vi "check_PVs_existed.vi"() -> ()   [LabVIEW 2013]
uses:
  <userlib>/caLab/Private/Get_PV-1D.vi
panel:
  out "Status":bool
  out "empty?":bool
  out "Numeric Control 2":i32
  out "1rst Value (string) 2":string[](array[string])
  out "Array 2":string[](array[string])
  out "Array":i32[](array[numeric])
  out "Numeric Control":i32
  out "sum":i16
  out "Error out":errorcluster
  out "size(s) 2":i32
  out "size(s)":i32
  out "1rst Value (string)":string[](array[string])
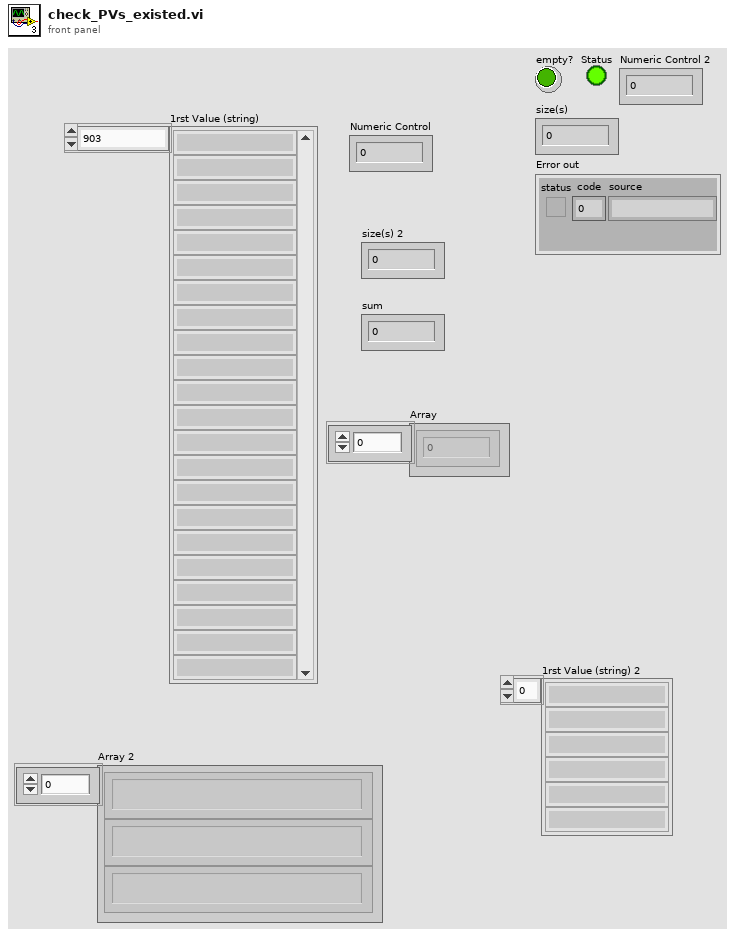
[diagram p1: front panel]
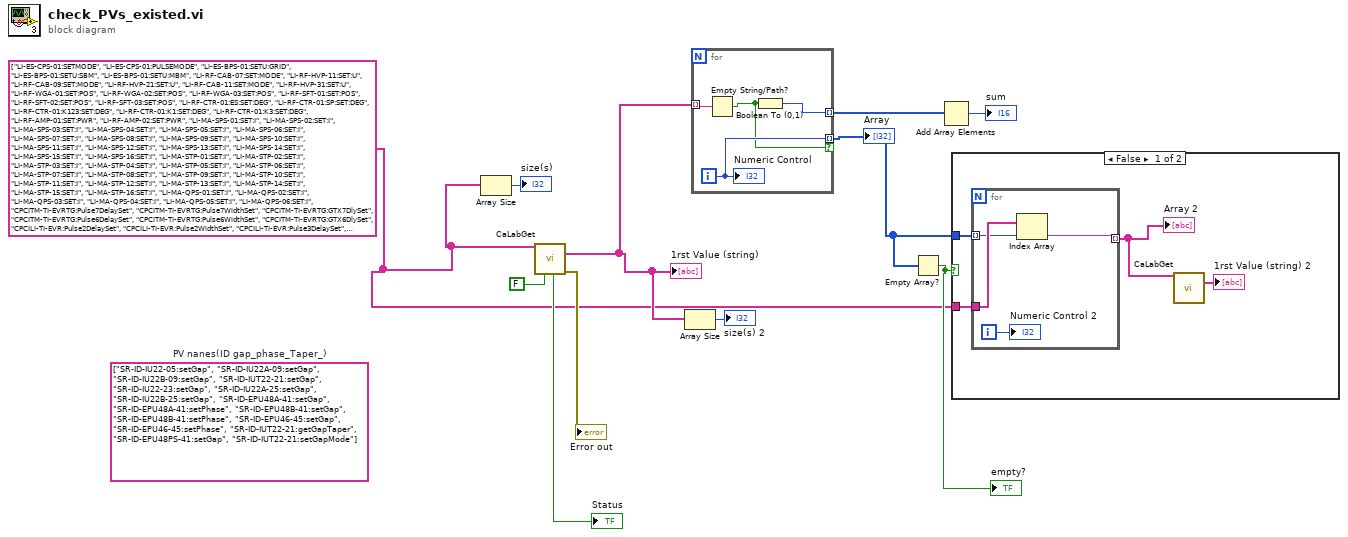
[diagram p0: block diagram]
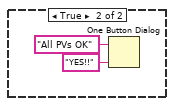
[diagram p2: hidden frame]
diagram:
  (unwired) string[] ["SR-ID-IU22-05:setGap", "SR-ID-IU22A-09:setGap", "SR-ID-IU22B-09:setGap", "SR-ID-IUT22-21:setGap", "SR-ID-IU22-23:setGap", "SR-ID-IU22A-25:setGap", "SR-ID-IU22B-25:setGap", "SR-ID-EPU48A-41:setGap", "SR-ID-EPU48A-41:setPhase", "SR-ID-EPU48B-41:setGap", "SR-ID-EPU48B-41:setPhase", "SR-ID-EPU46-45:setGap", "SR-ID-EPU46-45:setPhase", "SR-ID-IUT22-21:getGapTaper", "SR-ID-EPU48PS-41:setGap", "SR-ID-IUT22-21:setGapMode"]  # PV nanes(ID gap_phase_Taper_)
  w1 = string[] ["LI-ES-CPS-01:SETMODE", "LI-ES-CPS-01:PULSEMODE", "LI-ES-BPS-01:SETU:GRID", "LI-ES-BPS-01:SETU:SBM", "LI-ES-BPS-01:SETU:MBM", "LI-RF-CAB-07:SET:MODE", "LI-RF-HVP-11:SET:U", "LI-RF-CAB-09:SET:MODE", "LI-RF-HVP-21:SET:U", "LI-RF-CAB-11:SET:MODE", "LI-RF-HVP-31:SET:U", "LI-RF-WGA-01:SET:POS", "LI-RF-WGA-02:SET:POS", "LI-RF-WGA-03:SET:POS", "LI-RF-SFT-01:SET:POS", "LI-RF-SFT-02:SET:POS", "LI-RF-SFT-03:SET:POS", "LI-RF-CTR-01:ES:SET:DEG", "LI-RF-CTR-01:SP:SET:DEG", "LI-RF-CTR-01:K123:SET:DEG", "LI-RF-CTR-01:K1:SET:DEG", "LI-RF-CTR-01:K3:SET:DEG", "LI-RF-AMP-01:SET:PWR", "LI-RF-AMP-02:SET:PWR", "LI-MA-SPS-01:SET:I", "LI-MA-SPS-02:SET:I", "LI-MA-SPS-03:SET:I", "LI-MA-SPS-04:SET:I", "LI-MA-SPS-05:SET:I", "LI-MA-SPS-06:SET:I", "LI-MA-SPS-07:SET:I", "LI-MA-SPS-08:SET:I", "LI-MA-SPS-09:SET:I", "LI-MA-SPS-10:SET:I", "LI-MA-SPS-11:SET:I", "LI-MA-SPS-12:SET:I", "LI-MA-SPS-13:SET:I", "LI-MA-SPS-14:SET:I", "LI-MA-SPS-15:SET:I", "LI-MA-SPS-16:SET:I", "LI-MA-STP-01:SET:I", "LI-MA-STP-02:SET:I", "LI-MA-STP-03:SET:I", "LI-MA-STP-04:SET:I", "LI-MA-STP-05:SET:I", "LI-MA-STP-06:SET:I", "LI-MA-STP-07:SET:I", "LI-MA-STP-08:SET:I", "LI-MA-STP-09:SET:I", "LI-MA-STP-10:SET:I", "LI-MA-STP-11:SET:I", "LI-MA-STP-12:SET:I", "LI-MA-STP-13:SET:I", "LI-MA-STP-14:SET:I", "LI-MA-STP-15:SET:I", "LI-MA-STP-16:SET:I", "LI-MA-QPS-01:SET:I", "LI-MA-QPS-02:SET:I", "LI-MA-QPS-03:SET:I", "LI-MA-QPS-04:SET:I", "LI-MA-QPS-05:SET:I", "LI-MA-QPS-06:SET:I", "CPCITM-TI-EVRTG:Pulse7DelaySet", "CPCITM-TI-EVRTG:Pulse7WidthSet", "CPCITM-TI-EVRTG:GTX7DlySet", "CPCITM-TI-EVRTG:Pulse6DelaySet", "CPCITM-TI-EVRTG:Pulse6WidthSet", "CPCITM-TI-EVRTG:GTX6DlySet", "CPCILI-TI-EVR:Pulse2DelaySet", "CPCILI-TI-EVR:Pulse2WidthSet", "CPCILI-TI-EVR:Pulse3DelaySet", "CPCILI-TI-EVR:Pulse3WidthSet", "CPCILI-TI-EVR:Pulse4DelaySet", "CPCILI-TI-EVR:Pulse4WidthSet", "CPCILI-TI-EVR:Pulse5DelaySet", "CPCILI-TI-EVR:Pulse5WidthSet", "CPCILI-TI-EVR:Pulse6DelaySet", "CPCILI-TI-EVR:Pulse6WidthSet", "CPCILI-TI-EVR:Pulse7DelaySet", "CPCILI-TI-EVR:Pulse7WidthSet", "CPCILI-TI-EVR:Pulse8DelaySet", "CPCILI-TI-EVR:Pulse8WidthSet", "CPCILI-TI-EVR:Pulse9DelaySet", "CPCILI-TI-EVR:Pulse9WidthSet", "CPCITM-TI-EVRTG:GTX6DlySet", "CPCITM-TI-EVRTG:GTX7DlySet", "LTB-PS-HC-1:setI", "LTB-PS-HC-2:setI", "LTB-PS-HC-3:setI", "LTB-PS-HC-4:setI", "LTB-PS-HC-5:setI", "LTB-PS-VC-1:setI", "LTB-PS-VC-2:setI", "LTB-PS-VC-3:setI", "LTB-PS-VC-4:setI", "LTB-PS-VC-5:setI", "LTB-PS-VC-6:setI", "LTB-PS-VC-7:setI", "LTB-PS-Q1A:setI", "LTB-PS-Q1B:setI", "LTB-PS-Q1C:setI", "LTB-PS-Q2A:setI", "LTB-PS-Q2B:setI", "LTB-PS-Q2C:setI", "LTB-PS-Q3A:setI", "LTB-PS-Q3B:setI", "LTB-PS-Q4A:setI", "LTB-PS-Q4B:setI", "LTB-PS-QQ:setI", "LTB-PS-BEND-1:setI", "LTB-PS-VC-2a:setI", "LTB-PS-HC-3a:setI", "LTB-PS-HC-3b:setI", "LTB-PS-HC-4a:setI", "LTB-PS-HC-5a:setI", "LI-DI-SLIT-motor:axis2Position1", "LI-DI-SLIT-motor:axis1Position1", "BR-PS-HC-101:setI", "BR-PS-HC-102:setI", "BR-PS-HC-103:setI", "BR-PS-HC-104:setI", "BR-PS-HC-105:setI", "BR-PS-HC-106:setI", "BR-PS-HC-107:setI", "BR-PS-HC-108:setI", "BR-PS-HC-109:setI", "BR-PS-HC-110:setI", "BR-PS-HC-201:setI", "BR-PS-HC-202:setI", "BR-PS-HC-203:setI", "BR-PS-HC-204:setI", "BR-PS-HC-205:setI", "BR-PS-HC-206:setI", "BR-PS-HC-207:setI", "BR-PS-HC-208:setI", "BR-PS-HC-209:setI", "BR-PS-HC-210:setI", "BR-PS-HC-301:setI", "BR-PS-HC-302:setI", "BR-PS-HC-303:setI", "BR-PS-HC-304:setI", "BR-PS-HC-305:setI", "BR-PS-HC-306:setI", "BR-PS-HC-307:setI", "BR-PS-HC-308:setI", "BR-PS-HC-309:setI", "BR-PS-HC-310:setI", "BR-PS-HC-401:setI", "BR-PS-HC-402:setI", "BR-PS-HC-403:setI", "BR-PS-HC-404:setI", "BR-PS-HC-405:setI", "BR-PS-HC-406:setI", "BR-PS-HC-407:setI", "BR-PS-HC-408:setI", "BR-PS-HC-409:setI", "BR-PS-HC-410:setI", "BR-PS-HC-501:setI", "BR-PS-HC-502:setI", "BR-PS-HC-503:setI", "BR-PS-HC-504:setI", "BR-PS-HC-505:setI", "BR-PS-HC-506:setI", "BR-PS-HC-507:setI", "BR-PS-HC-508:setI", "BR-PS-HC-509:setI", "BR-PS-HC-510:setI", "BR-PS-HC-601:setI", "BR-PS-HC-602:setI", "BR-PS-HC-603:setI", "BR-PS-HC-603a:setI", "BR-PS-HC-604:setI", "BR-PS-HC-605:setI", "BR-PS-HC-606:setI", "BR-PS-HC-606a:setI", "BR-PS-HC-607:setI", "BR-PS-HC-608:setI", "BR-PS-HC-609:setI", "BR-PS-HC-610:setI", "BR-PS-VC-101:setI", "BR-PS-VC-102:setI", "BR-PS-VC-103:setI", "BR-PS-VC-104:setI", "BR-PS-VC-105:setI", "BR-PS-VC-106:setI", "BR-PS-VC-201:setI", "BR-PS-VC-202:setI", "BR-PS-VC-203:setI", "BR-PS-VC-204:setI", "BR-PS-VC-205:setI", "BR-PS-VC-206:setI", "BR-PS-VC-301:setI", "BR-PS-VC-302:setI", "BR-PS-VC-303:setI", "BR-PS-VC-304:setI", "BR-PS-VC-305:setI", "BR-PS-VC-306:setI", "BR-PS-VC-401:setI", "BR-PS-VC-402:setI", "BR-PS-VC-403:setI", "BR-PS-VC-404:setI", "BR-PS-VC-405:setI", "BR-PS-VC-406:setI", "BR-PS-VC-501:setI", "BR-PS-VC-502:setI", "BR-PS-VC-503:setI", "BR-PS-VC-504:setI", "BR-PS-VC-505:setI", "BR-PS-VC-506:setI", "BR-PS-VC-601:setI", "BR-PS-VC-602:setI", "BR-PS-VC-602a:setI", "BR-PS-VC-603:setI", "BR-PS-VC-604:setI", "BR-PS-VC-604a:setI", "BR-PS-VC-605:setI", "BR-PS-VC-606:setI", "BR-PS-VC-100a:setI", "BR-PS-SD:setI", "BR-PS-SF:setI", "cpsc_027:AO:SLOW_SET:CH:1", "cpsc_037:AO:SLOW_SET:CH:3", "BR-RF-LLRF:setStationPhase", "TI-INJ-PROC:setTinj", "BR-PS-INJ-SE:setHV", "CPCIPM-TI-EVR:Pulse1DelaySet", "BR-PS-INJ-KI:setHV", "CPCIPM-TI-EVR:Pulse2DelaySet", "BR-PS-QF:setWfDC", "BR-PS-QM:setWfDC", "BR-PS-Q1:setWfDC", "BR-PS-Q2:setWfDC", "BR-PS-BEND:setWfDC", "BTS-PS-HC-1:setI", "BTS-PS-HC-2:setI", "BTS-PS-HC-3:setI", "BTS-PS-HC-4:setI", "BTS-PS-HC-5:setI", "BTS-PS-VC-2:setI", "BTS-PS-VC-3:setI", "BTS-PS-VC-4:setI", "BTS-PS-VC-5:setI", "BTS-PS-VC-6:setI", "BTS-PS-Q1A:setI", "BTS-PS-Q1B:setI", "BTS-PS-Q1C:setI", "BTS-PS-Q2A:setI", "BTS-PS-Q2B:setI", "BTS-PS-Q2C:setI", "BTS-PS-Q3A:setI", "BTS-PS-BEND-1:setI", "BTS-PS-BEND-2:setI", "BR-PS-EXT-K1:setHV", "BR-PS-EXT-K2:setHV", "SR-PS-INJ-SE1:setHV", "SR-PS-INJ-SE2:setHV", "SR-PS-INJ-K1:setHV", "SR-PS-INJ-K2:setHV", "SR-PS-INJ-K3:setHV", "SR-PS-INJ-K4:setHV", "CPCIPM-TI-EVR:Pulse4DelaySet", "CPCIPM-TI-EVR:Pulse5DelaySet", "CPCIPM-TI-EVR:Pulse3DelaySet", "CPCIPM-TI-EVR:Pulse6DelaySet", "CPCIPM-TI-EVR:Pulse7DelaySet", "T560:setADelay", "T560:setBDelay", "T560:setCDelay", "T560:setDDelay", "CPCIPM-TI-EVR:Pulse4DelaySet", "CPCIPM-TI-EVR:Pulse5DelaySet", "BR-PS-EXT-SE1:setHV", "BR-PS-EXT-SE2:setHV", "CPCIPM-TI-EVR:Pulse3DelaySet", "CPCIPM-TI-EVR:Pulse11DelaySet", "SR-PS-BEND:setI", "SR-PS-HC-011:setI", "SR-PS-HC-012:setI", "SR-PS-HC-013:setI", "SR-PS-HC-014:setI", "SR-PS-HC-015:setI", "SR-PS-HC-016:setI", "SR-PS-HC-017:setI", "SR-PS-HC-021:setI", "SR-PS-HC-022:setI", "SR-PS-HC-023:setI", "SR-PS-HC-024:setI", "SR-PS-HC-025:setI", "SR-PS-HC-026:setI", "SR-PS-HC-027:setI", "SR-PS-HC-031:setI", "SR-PS-HC-032:setI", "SR-PS-HC-033:setI", "SR-PS-HC-034:setI", "SR-PS-HC-035:setI", "SR-PS-HC-036:setI", "SR-PS-HC-037:setI", "SR-PS-HC-041:setI", "SR-PS-HC-042:setI", "SR-PS-HC-043:setI", "SR-PS-HC-044:setI", "SR-PS-HC-045:setI", "SR-PS-HC-046:setI", "SR-PS-HC-047:setI", "SR-PS-HC-051:setI", "SR-PS-HC-052:setI", "SR-PS-HC-053:setI", "SR-PS-HC-054:setI", "SR-PS-HC-055:setI", "SR-PS-HC-056:setI", "SR-PS-HC-057:setI", "SR-PS-HC-061:setI", "SR-PS-HC-062:setI", "SR-PS-HC-063:setI", "SR-PS-HC-064:setI", "SR-PS-HC-065:setI", "SR-PS-HC-066:setI", "SR-PS-HC-067:setI", "SR-PS-HC-071:setI", "SR-PS-HC-072:setI", "SR-PS-HC-073:setI", "SR-PS-HC-074:setI", "SR-PS-HC-075:setI", "SR-PS-HC-076:setI", "SR-PS-HC-077:setI", "SR-PS-HC-081:setI", "SR-PS-HC-082:setI", "SR-PS-HC-083:setI", "SR-PS-HC-084:setI", "SR-PS-HC-085:setI", "SR-PS-HC-086:setI", "SR-PS-HC-087:setI", "SR-PS-HC-091:setI", "SR-PS-HC-092:setI", "SR-PS-HC-093:setI", "SR-PS-HC-094:setI", "SR-PS-HC-095:setI", "SR-PS-HC-096:setI", "SR-PS-HC-097:setI", "SR-PS-HC-101:setI", "SR-PS-HC-102:setI", "SR-PS-HC-103:setI", "SR-PS-HC-104:setI", "SR-PS-HC-105:setI", "SR-PS-HC-106:setI", "SR-PS-HC-107:setI", "SR-PS-HC-111:setI", "SR-PS-HC-112:setI", "SR-PS-HC-113:setI", "SR-PS-HC-114:setI", "SR-PS-HC-115:setI", "SR-PS-HC-116:setI", "SR-PS-HC-117:setI", "SR-PS-HC-121:setI", "SR-PS-HC-122:setI", "SR-PS-HC-123:setI", "SR-PS-HC-124:setI", "SR-PS-HC-125:setI", "SR-PS-HC-126:setI", "SR-PS-HC-127:setI", "SR-PS-HC-131:setI", "SR-PS-HC-132:setI", "SR-PS-HC-133:setI", "SR-PS-HC-134:setI", "SR-PS-HC-135:setI", "SR-PS-HC-136:setI", "SR-PS-HC-137:setI", "SR-PS-HC-141:setI", "SR-PS-HC-142:setI", "SR-PS-HC-143:setI", "SR-PS-HC-144:setI", "SR-PS-HC-145:setI", "SR-PS-HC-146:setI", "SR-PS-HC-147:setI", "SR-PS-HC-151:setI", "SR-PS-HC-152:setI", "SR-PS-HC-153:setI", "SR-PS-HC-154:setI", "SR-PS-HC-155:setI", "SR-PS-HC-156:setI", "SR-PS-HC-157:setI", "SR-PS-HC-161:setI", "SR-PS-HC-162:setI", "SR-PS-HC-163:setI", "SR-PS-HC-164:setI", "SR-PS-HC-165:setI", "SR-PS-HC-166:setI", "SR-PS-HC-167:setI", "SR-PS-HC-171:setI", "SR-PS-HC-172:setI", "SR-PS-HC-173:setI", "SR-PS-HC-174:setI", "SR-PS-HC-175:setI", "SR-PS-HC-176:setI", "SR-PS-HC-177:setI", "SR-PS-HC-181:setI", "SR-PS-HC-182:setI", "SR-PS-HC-183:setI", "SR-PS-HC-184:setI", "SR-PS-HC-185:setI", "SR-PS-HC-186:setI", "SR-PS-HC-187:setI", "SR-PS-HC-191:setI", "SR-PS-HC-192:setI", "SR-PS-HC-193:setI", "SR-PS-HC-194:setI", "SR-PS-HC-195:setI", "SR-PS-HC-196:setI", "SR-PS-HC-197:setI", "SR-PS-HC-201:setI", "SR-PS-HC-202:setI", "SR-PS-HC-203:setI", "SR-PS-HC-204:setI", "SR-PS-HC-205:setI", "SR-PS-HC-206:setI", "SR-PS-HC-207:setI", "SR-PS-HC-211:setI", "SR-PS-HC-212:setI", "SR-PS-HC-213:setI", "SR-PS-HC-214:setI", "SR-PS-HC-215:setI", "SR-PS-HC-216:setI", "SR-PS-HC-217:setI", "SR-PS-HC-221:setI", "SR-PS-HC-222:setI", "SR-PS-HC-223:setI", "SR-PS-HC-224:setI", "SR-PS-HC-225:setI", "SR-PS-HC-226:setI", "SR-PS-HC-227:setI", "SR-PS-HC-231:setI", "SR-PS-HC-232:setI", "SR-PS-HC-233:setI", "SR-PS-HC-234:setI", "SR-PS-HC-235:setI", "SR-PS-HC-236:setI", "SR-PS-HC-237:setI", "SR-PS-HC-241:setI", "SR-PS-HC-242:setI", "SR-PS-HC-243:setI", "SR-PS-HC-244:setI", "SR-PS-HC-245:setI", "SR-PS-HC-246:setI", "SR-PS-HC-247:setI", "SR-PS-VC-011:setI", "SR-PS-VC-012:setI", "SR-PS-VC-013:setI", "SR-PS-VC-014:setI", "SR-PS-VC-015:setI", "SR-PS-VC-016:setI", "SR-PS-VC-017:setI", "SR-PS-VC-021:setI", "SR-PS-VC-022:setI", "SR-PS-VC-023:setI", "SR-PS-VC-024:setI", "SR-PS-VC-025:setI", "SR-PS-VC-026:setI", "SR-PS-VC-027:setI", "SR-PS-VC-031:setI", "SR-PS-VC-032:setI", "SR-PS-VC-033:setI", "SR-PS-VC-034:setI", "SR-PS-VC-035:setI", "SR-PS-VC-036:setI", "SR-PS-VC-037:setI", "SR-PS-VC-041:setI", "SR-PS-VC-042:setI", "SR-PS-VC-043:setI", "SR-PS-VC-044:setI", "SR-PS-VC-045:setI", "SR-PS-VC-046:setI", "SR-PS-VC-047:setI", "SR-PS-VC-051:setI", "SR-PS-VC-052:setI", "SR-PS-VC-053:setI", "SR-PS-VC-054:setI", "SR-PS-VC-055:setI", "SR-PS-VC-056:setI", "SR-PS-VC-057:setI", "SR-PS-VC-061:setI", "SR-PS-VC-062:setI", "SR-PS-VC-063:setI", "SR-PS-VC-064:setI", "SR-PS-VC-065:setI", "SR-PS-VC-066:setI", "SR-PS-VC-067:setI", "SR-PS-VC-071:setI", "SR-PS-VC-072:setI", "SR-PS-VC-073:setI", "SR-PS-VC-074:setI", "SR-PS-VC-075:setI", "SR-PS-VC-076:setI", "SR-PS-VC-077:setI", "SR-PS-VC-081:setI", "SR-PS-VC-082:setI", "SR-PS-VC-083:setI", "SR-PS-VC-084:setI", "SR-PS-VC-085:setI", "SR-PS-VC-086:setI", "SR-PS-VC-087:setI", "SR-PS-VC-091:setI", "SR-PS-VC-092:setI", "SR-PS-VC-093:setI", "SR-PS-VC-094:setI", "SR-PS-VC-095:setI", "SR-PS-VC-096:setI", "SR-PS-VC-097:setI", "SR-PS-VC-101:setI", "SR-PS-VC-102:setI", "SR-PS-VC-103:setI", "SR-PS-VC-104:setI", "SR-PS-VC-105:setI", "SR-PS-VC-106:setI", "SR-PS-VC-107:setI", "SR-PS-VC-111:setI", "SR-PS-VC-112:setI", "SR-PS-VC-113:setI", "SR-PS-VC-114:setI", "SR-PS-VC-115:setI", "SR-PS-VC-116:setI", "SR-PS-VC-117:setI", "SR-PS-VC-121:setI", "SR-PS-VC-122:setI", "SR-PS-VC-123:setI", "SR-PS-VC-124:setI", "SR-PS-VC-125:setI", "SR-PS-VC-126:setI", "SR-PS-VC-127:setI", "SR-PS-VC-131:setI", "SR-PS-VC-132:setI", "SR-PS-VC-133:setI", "SR-PS-VC-134:setI", "SR-PS-VC-135:setI", "SR-PS-VC-136:setI", "SR-PS-VC-137:setI", "SR-PS-VC-141:setI", "SR-PS-VC-142:setI", "SR-PS-VC-143:setI", "SR-PS-VC-144:setI", "SR-PS-VC-145:setI", "SR-PS-VC-146:setI", "SR-PS-VC-147:setI", "SR-PS-VC-151:setI", "SR-PS-VC-152:setI", "SR-PS-VC-153:setI", "SR-PS-VC-154:setI", "SR-PS-VC-155:setI", "SR-PS-VC-156:setI", "SR-PS-VC-157:setI", "SR-PS-VC-161:setI", "SR-PS-VC-162:setI", "SR-PS-VC-163:setI", "SR-PS-VC-164:setI", "SR-PS-VC-165:setI", "SR-PS-VC-166:setI", "SR-PS-VC-167:setI", "SR-PS-VC-171:setI", "SR-PS-VC-172:setI", "SR-PS-VC-173:setI", "SR-PS-VC-174:setI", "SR-PS-VC-175:setI", "SR-PS-VC-176:setI", "SR-PS-VC-177:setI", "SR-PS-VC-181:setI", "SR-PS-VC-182:setI", "SR-PS-VC-183:setI", "SR-PS-VC-184:setI", "SR-PS-VC-185:setI", "SR-PS-VC-186:setI", "SR-PS-VC-187:setI", "SR-PS-VC-191:setI", "SR-PS-VC-192:setI", "SR-PS-VC-193:setI", "SR-PS-VC-194:setI", "SR-PS-VC-195:setI", "SR-PS-VC-196:setI", "SR-PS-VC-197:setI", "SR-PS-VC-201:setI", "SR-PS-VC-202:setI", "SR-PS-VC-203:setI", "SR-PS-VC-204:setI", "SR-PS-VC-205:setI", "SR-PS-VC-206:setI", "SR-PS-VC-207:setI", "SR-PS-VC-211:setI", "SR-PS-VC-212:setI", "SR-PS-VC-213:setI", "SR-PS-VC-214:setI", "SR-PS-VC-215:setI", "SR-PS-VC-216:setI", "SR-PS-VC-217:setI", "SR-PS-VC-221:setI", "SR-PS-VC-222:setI", "SR-PS-VC-223:setI", "SR-PS-VC-224:setI", "SR-PS-VC-225:setI", "SR-PS-VC-226:setI", "SR-PS-VC-227:setI", "SR-PS-VC-231:setI", "SR-PS-VC-232:setI", "SR-PS-VC-233:setI", "SR-PS-VC-234:setI", "SR-PS-VC-235:setI", "SR-PS-VC-236:setI", "SR-PS-VC-237:setI", "SR-PS-VC-241:setI", "SR-PS-VC-242:setI", "SR-PS-VC-243:setI", "SR-PS-VC-244:setI", "SR-PS-VC-245:setI", "SR-PS-VC-246:setI", "SR-PS-VC-247:setI", "SR-PS-QL1-0101:setI", "SR-PS-QL2-0102:setI", "SR-PS-QL3-0103:setI", "SR-PS-QS4-0104:setI", "SR-PS-QS5-0105:setI", "SR-PS-QS5-0106:setI", "SR-PS-QS4-0107:setI", "SR-PS-QS3-0108:setI", "SR-PS-QS2-0109:setI", "SR-PS-QS1-0110:setI", "SR-PS-QS1-0201:setI", "SR-PS-QS2-0202:setI", "SR-PS-QS3-0203:setI", "SR-PS-QS4-0204:setI", "SR-PS-QS5-0205:setI", "SR-PS-QS5-0206:setI", "SR-PS-QS4-0207:setI", "SR-PS-QS3-0208:setI", "SR-PS-QS2-0209:setI", "SR-PS-QS1-0210:setI", "SR-PS-QS1-0301:setI", "SR-PS-QS2-0302:setI", "SR-PS-QS3-0303:setI", "SR-PS-QS4-0304:setI", "SR-PS-QS5-0305:setI", "SR-PS-QS5-0306:setI", "SR-PS-QS4-0307:setI", "SR-PS-QS3-0308:setI", "SR-PS-QS2-0309:setI", "SR-PS-QS1-0310:setI", "SR-PS-QS1-0401:setI", "SR-PS-QS2-0402:setI", "SR-PS-QS3-0403:setI", "SR-PS-QS4-0404:setI", "SR-PS-QS5-0405:setI", "SR-PS-QS5-0406:setI", "SR-PS-QS4-0407:setI", "SR-PS-QL3-0408:setI", "SR-PS-QL2-0409:setI", "SR-PS-QL1-0410:setI", "SR-PS-QL1-0501:setI", "SR-PS-QL2-0502:setI", "SR-PS-QL3-0503:setI", "SR-PS-QS4-0504:setI", "SR-PS-QS5-0505:setI", "SR-PS-QS5-0506:setI", "SR-PS-QS4-0507:setI", "SR-PS-QS3-0508:setI", "SR-PS-QS2-0509:setI", "SR-PS-QS1-0510:setI", "SR-PS-QS1-0601:setI", "SR-PS-QS2-0602:setI", "SR-PS-QS3-0603:setI", "SR-PS-QS4-0604:setI", "SR-PS-QS5-0605:setI", "SR-PS-QS5-0606:setI", "SR-PS-QS4-0607:setI", "SR-PS-QS3-0608:setI", "SR-PS-QS2-0609:setI", "SR-PS-QS1-0610:setI", "SR-PS-QS1-0701:setI", "SR-PS-QS2-0702:setI", "SR-PS-QS3-0703:setI", "SR-PS-QS4-0704:setI", "SR-PS-QS5-0705:setI", "SR-PS-QS5-0706:setI", "SR-PS-QS4-0707:setI", "SR-PS-QS3-0708:setI", "SR-PS-QS2-0709:setI", "SR-PS-QS1-0710:setI", "SR-PS-QS1-0801:setI", "SR-PS-QS2-0802:setI", "SR-PS-QS3-0803:setI", "SR-PS-QS4-0804:setI", "SR-PS-QS5-0805:setI", "SR-PS-QS5-0806:setI", "SR-PS-QS4-0807:setI", "SR-PS-QL3-0808:setI", "SR-PS-QL2-0809:setI", "SR-PS-QL1-0810:setI", "SR-PS-QL1-0901:setI", "SR-PS-QL2-0902:setI", "SR-PS-QL3-0903:setI", "SR-PS-QS4-0904:setI", "SR-PS-QS5-0905:setI", "SR-PS-QS5-0906:setI", "SR-PS-QS4-0907:setI", "SR-PS-QS3-0908:setI", "SR-PS-QS2-0909:setI", "SR-PS-QS1-0910:setI", "SR-PS-QS1-1001:setI", "SR-PS-QS2-1002:setI", "SR-PS-QS3-1003:setI", "SR-PS-QS4-1004:setI", "SR-PS-QS5-1005:setI", "SR-PS-QS5-1006:setI", "SR-PS-QS4-1007:setI", "SR-PS-QS3-1008:setI", "SR-PS-QS2-1009:setI", "SR-PS-QS1-1010:setI", "SR-PS-QS1-1101:setI", "SR-PS-QS2-1102:setI", "SR-PS-QS3-1103:setI", "SR-PS-QS4-1104:setI", "SR-PS-QS5-1105:setI", "SR-PS-QS5-1106:setI", "SR-PS-QS4-1107:setI", "SR-PS-QS3-1108:setI", "SR-PS-QS2-1109:setI", "SR-PS-QS1-1110:setI", "SR-PS-QS1-1201:setI", "SR-PS-QS2-1202:setI", "SR-PS-QS3-1203:setI", "SR-PS-QS4-1204:setI", "SR-PS-QS5-1205:setI", "SR-PS-QS5-1206:setI", "SR-PS-QS4-1207:setI", "SR-PS-QL3-1208:setI", "SR-PS-QL2-1209:setI", "SR-PS-QL1-1210:setI", "SR-PS-QL1-1301:setI", "SR-PS-QL2-1302:setI", "SR-PS-QL3-1303:setI", "SR-PS-QS4-1304:setI", "SR-PS-QS5-1305:setI", "SR-PS-QS5-1306:setI", "SR-PS-QS4-1307:setI", "SR-PS-QS3-1308:setI", "SR-PS-QS2-1309:setI", "SR-PS-QS1-1310:setI", "SR-PS-QS1-1401:setI", "SR-PS-QS2-1402:setI", "SR-PS-QS3-1403:setI", "SR-PS-QS4-1404:setI", "SR-PS-QS5-1405:setI", "SR-PS-QS5-1406:setI", "SR-PS-QS4-1407:setI", "SR-PS-QS3-1408:setI", "SR-PS-QS2-1409:setI", "SR-PS-QS1-1410:setI", "SR-PS-QS1-1501:setI", "SR-PS-QS2-1502:setI", "SR-PS-QS3-1503:setI", "SR-PS-QS4-1504:setI", "SR-PS-QS5-1505:setI", "SR-PS-QS5-1506:setI", "SR-PS-QS4-1507:setI", "SR-PS-QS3-1508:setI", "SR-PS-QS2-1509:setI", "SR-PS-QS1-1510:setI", "SR-PS-QS1-1601:setI", "SR-PS-QS2-1602:setI", "SR-PS-QS3-1603:setI", "SR-PS-QS4-1604:setI", "SR-PS-QS5-1605:setI", "SR-PS-QS5-1606:setI", "SR-PS-QS4-1607:setI", "SR-PS-QL3-1608:setI", "SR-PS-QL2-1609:setI", "SR-PS-QL1-1610:setI", "SR-PS-QL1-1701:setI", "SR-PS-QL2-1702:setI", "SR-PS-QL3-1703:setI", "SR-PS-QS4-1704:setI", "SR-PS-QS5-1705:setI", "SR-PS-QS5-1706:setI", "SR-PS-QS4-1707:setI", "SR-PS-QS3-1708:setI", "SR-PS-QS2-1709:setI", "SR-PS-QS1-1710:setI", "SR-PS-QS1-1801:setI", "SR-PS-QS2-1802:setI", "SR-PS-QS3-1803:setI", "SR-PS-QS4-1804:setI", "SR-PS-QS5-1805:setI", "SR-PS-QS5-1806:setI", "SR-PS-QS4-1807:setI", "SR-PS-QS3-1808:setI", "SR-PS-QS2-1809:setI", "SR-PS-QS1-1810:setI", "SR-PS-QS1-1901:setI", "SR-PS-QS2-1902:setI", "SR-PS-QS3-1903:setI", "SR-PS-QS4-1904:setI", "SR-PS-QS5-1905:setI", "SR-PS-QS5-1906:setI", "SR-PS-QS4-1907:setI", "SR-PS-QS3-1908:setI", "SR-PS-QS2-1909:setI", "SR-PS-QS1-1910:setI", "SR-PS-QS1-2001:setI", "SR-PS-QS2-2002:setI", "SR-PS-QS3-2003:setI", "SR-PS-QS4-2004:setI", "SR-PS-QS5-2005:setI", "SR-PS-QS5-2006:setI", "SR-PS-QS4-2007:setI", "SR-PS-QL3-2008:setI", "SR-PS-QL2-2009:setI", "SR-PS-QL1-2010:setI", "SR-PS-QL1-2101:setI", "SR-PS-QL2-2102:setI", "SR-PS-QL3-2103:setI", "SR-PS-QS4-2104:setI", "SR-PS-QS5-2105:setI", "SR-PS-QS5-2106:setI", "SR-PS-QS4-2107:setI", "SR-PS-QS3-2108:setI", "SR-PS-QS2-2109:setI", "SR-PS-QS1-2110:setI", "SR-PS-QS1-2201:setI", "SR-PS-QS2-2202:setI", "SR-PS-QS3-2203:setI", "SR-PS-QS4-2204:setI", "SR-PS-QS5-2205:setI", "SR-PS-QS5-2206:setI", "SR-PS-QS4-2207:setI", "SR-PS-QS3-2208:setI", "SR-PS-QS2-2209:setI", "SR-PS-QS1-2210:setI", "SR-PS-QS1-2301:setI", "SR-PS-QS2-2302:setI", "SR-PS-QS3-2303:setI", "SR-PS-QS4-2304:setI", "SR-PS-QS5-2305:setI", "SR-PS-QS5-2306:setI", "SR-PS-QS4-2307:setI", "SR-PS-QS3-2308:setI", "SR-PS-QS2-2309:setI", "SR-PS-QS1-2310:setI", "SR-PS-QS1-2401:setI", "SR-PS-QS2-2402:setI", "SR-PS-QS3-2403:setI", "SR-PS-QS4-2404:setI", "SR-PS-QS5-2405:setI", "SR-PS-QS5-2406:setI", "SR-PS-QS4-2407:setI", "SR-PS-QL3-2408:setI", "SR-PS-QL2-2409:setI", "SR-PS-QL1-2410:setI", "SR-PS-S1-011:setI", "SR-PS-S2-012:setI", "SR-PS-SD-013:setI", "SR-PS-SF-014:setI", "SR-PS-SD-015:setI", "SR-PS-S4-016:setI", "SR-PS-S3-017:setI", "SR-PS-S5-021:setI", "SR-PS-S6-022:setI", "SR-PS-SD-023:setI", "SR-PS-SF-024:setI", "SR-PS-SD-025:setI", "SR-PS-S6-026:setI", "SR-PS-S5-027:setI", "SR-PS-S5-031:setI", "SR-PS-S6-032:setI", "SR-PS-SD-033:setI", "SR-PS-SF-034:setI", "SR-PS-SD-035:setI", "SR-PS-S6-036:setI", "SR-PS-S5-037:setI", "SR-PS-S3-041:setI", "SR-PS-S4-042:setI", "SR-PS-SD-043:setI", "SR-PS-SF-044:setI", "SR-PS-SD-045:setI", "SR-PS-S2-046:setI", "SR-PS-S1-047:setI", "SR-PS-S1-051:setI", "SR-PS-S2-052:setI", "SR-PS-SD-053:setI", "SR-PS-SF-054:setI", "SR-PS-SD-055:setI", "SR-PS-S4-056:setI", "SR-PS-S3-057:setI", "SR-PS-S5-061:setI", "SR-PS-S6-062:setI", "SR-PS-SD-063:setI", "SR-PS-SF-064:setI", "SR-PS-SD-065:setI", "SR-PS-S6-066:setI", "SR-PS-S5-067:setI", "SR-PS-S5-071:setI", "SR-PS-S6-072:setI", "SR-PS-SD-073:setI", "SR-PS-SF-074:setI", "SR-PS-SD-075:setI", "SR-PS-S6-076:setI", "SR-PS-S5-077:setI", "SR-PS-S3-081:setI", "SR-PS-S4-082:setI", "SR-PS-SD-083:setI", "SR-PS-SF-084:setI", "SR-PS-SD-085:setI", "SR-PS-S2-086:setI", "SR-PS-S1-087:setI", "SR-PS-S1-091:setI", "SR-PS-S2-092:setI", "SR-PS-SD-093:setI", "SR-PS-SF-094:setI", "SR-PS-SD-095:setI", "SR-PS-S4-096:setI", "SR-PS-S3-097:setI", "SR-PS-S5-101:setI", "SR-PS-S6-102:setI", "SR-PS-SD-103:setI", "SR-PS-SF-104:setI", "SR-PS-SD-105:setI", "SR-PS-S6-106:setI", "SR-PS-S5-107:setI", "SR-PS-S5-111:setI", "SR-PS-S6-112:setI", "SR-PS-SD-113:setI", "SR-PS-SF-114:setI", "SR-PS-SD-115:setI", "SR-PS-S6-116:setI", "SR-PS-S5-117:setI", "SR-PS-S3-121:setI", "SR-PS-S4-122:setI", "SR-PS-SD-123:setI", "SR-PS-SF-124:setI", "SR-PS-SD-125:setI", "SR-PS-S2-126:setI", "SR-PS-S1-127:setI", "SR-PS-S1-131:setI", "SR-PS-S2-132:setI", "SR-PS-SD-133:setI", "SR-PS-SF-134:setI", "SR-PS-SD-135:setI", "SR-PS-S4-136:setI", "SR-PS-S3-137:setI", "SR-PS-S5-141:setI", "SR-PS-S6-142:setI", "SR-PS-SD-143:setI", "SR-PS-SF-144:setI", "SR-PS-SD-145:setI", "SR-PS-S6-146:setI", "SR-PS-S5-147:setI", "SR-PS-S5-151:setI", "SR-PS-S6-152:setI", "SR-PS-SD-153:setI", "SR-PS-SF-154:setI", "SR-PS-SD-155:setI", "SR-PS-S6-156:setI", "SR-PS-S5-157:setI", "SR-PS-S3-161:setI", "SR-PS-S4-162:setI", "SR-PS-SD-163:setI", "SR-PS-SF-164:setI", "SR-PS-SD-165:setI", "SR-PS-S2-166:setI", "SR-PS-S1-167:setI", "SR-PS-S1-171:setI", "SR-PS-S2-172:setI", "SR-PS-SD-173:setI", "SR-PS-SF-174:setI", "SR-PS-SD-175:setI", "SR-PS-S4-176:setI", "SR-PS-S3-177:setI", "SR-PS-S5-181:setI", "SR-PS-S6-182:setI", "SR-PS-SD-183:setI", "SR-PS-SF-184:setI", "SR-PS-SD-185:setI", "SR-PS-S6-186:setI", "SR-PS-S5-187:setI", "SR-PS-S5-191:setI", "SR-PS-S6-192:setI", "SR-PS-SD-193:setI", "SR-PS-SF-194:setI", "SR-PS-SD-195:setI", "SR-PS-S6-196:setI", "SR-PS-S5-197:setI", "SR-PS-S3-201:setI", "SR-PS-S4-202:setI", "SR-PS-SD-203:setI", "SR-PS-SF-204:setI", "SR-PS-SD-205:setI", "SR-PS-S2-206:setI", "SR-PS-S1-207:setI", "SR-PS-S1-211:setI", "SR-PS-S2-212:setI", "SR-PS-SD-213:setI", "SR-PS-SF-214:setI", "SR-PS-SD-215:setI", "SR-PS-S4-216:setI", "SR-PS-S3-217:setI", "SR-PS-S5-221:setI", "SR-PS-S6-222:setI", "SR-PS-SD-223:setI", "SR-PS-SF-224:setI", "SR-PS-SD-225:setI", "SR-PS-S6-226:setI", "SR-PS-S5-227:setI", "SR-PS-S5-231:setI", "SR-PS-S6-232:setI", "SR-PS-SD-233:setI", "SR-PS-SF-234:setI", "SR-PS-SD-235:setI", "SR-PS-S6-236:setI", "SR-PS-S5-237:setI", "SR-PS-S3-241:setI", "SR-PS-S4-242:setI", "SR-PS-SD-243:setI", "SR-PS-SF-244:setI", "SR-PS-SD-245:setI", "SR-PS-S2-246:setI", "SR-PS-S1-247:setI", "SR-PS-SKEW-011:setI", "SR-PS-SKEW-012:setI", "SR-PS-SKEW-013:setI", "SR-PS-SKEW-014:setI", "SR-PS-SKEW-015:setI", "SR-PS-SKEW-016:setI", "SR-PS-SKEW-017:setI", "SR-PS-SKEW-021:setI", "SR-PS-SKEW-022:setI", "SR-PS-SKEW-023:setI", "SR-PS-SKEW-024:setI", "SR-PS-SKEW-025:setI", "SR-PS-SKEW-026:setI", "SR-PS-SKEW-027:setI", "SR-PS-SKEW-031:setI", "SR-PS-SKEW-032:setI", "SR-PS-SKEW-033:setI", "SR-PS-SKEW-034:setI", "SR-PS-SKEW-035:setI", "SR-PS-SKEW-036:setI", "SR-PS-SKEW-037:setI", "SR-PS-SKEW-041:setI", "SR-PS-SKEW-042:setI", "SR-PS-SKEW-043:setI", "SR-PS-SKEW-044:setI", "SR-PS-SKEW-045:setI", "SR-PS-SKEW-046:setI", "SR-PS-SKEW-047:setI", "SR-PS-SKEW-051:setI", "SR-PS-SKEW-052:setI", "SR-PS-SKEW-053:setI", "SR-PS-SKEW-054:setI", "SR-PS-SKEW-055:setI", "SR-PS-SKEW-056:setI", "SR-PS-SKEW-057:setI", "SR-PS-SKEW-061:setI", "SR-PS-SKEW-062:setI", "SR-PS-SKEW-063:setI", "SR-PS-SKEW-064:setI", "SR-PS-SKEW-065:setI", "SR-PS-SKEW-066:setI", "SR-PS-SKEW-067:setI", "SR-PS-SKEW-071:setI", "SR-PS-SKEW-072:setI", "SR-PS-SKEW-073:setI", "SR-PS-SKEW-074:setI", "SR-PS-SKEW-075:setI", "SR-PS-SKEW-076:setI", "SR-PS-SKEW-077:setI", "SR-PS-SKEW-081:setI", "SR-PS-SKEW-082:setI", "SR-PS-SKEW-083:setI", "SR-PS-SKEW-084:setI", "SR-PS-SKEW-085:setI", "SR-PS-SKEW-086:setI", "SR-PS-SKEW-087:setI", "SR-PS-SKEW-091:setI", "SR-PS-SKEW-092:setI", "SR-PS-SKEW-093:setI", "SR-PS-SKEW-094:setI", "SR-PS-SKEW-095:setI", "SR-PS-SKEW-096:setI", "SR-PS-SKEW-097:setI", "SR-PS-SKEW-101:setI", "SR-PS-SKEW-102:setI", "SR-PS-SKEW-103:setI", "SR-PS-SKEW-104:setI", "SR-PS-SKEW-105:setI", "SR-PS-SKEW-106:setI", "SR-PS-SKEW-107:setI", "SR-PS-SKEW-111:setI", "SR-PS-SKEW-112:setI", "SR-PS-SKEW-113:setI", "SR-PS-SKEW-114:setI", "SR-PS-SKEW-115:setI", "SR-PS-SKEW-116:setI", "SR-PS-SKEW-117:setI", "SR-PS-SKEW-121:setI", "SR-PS-SKEW-122:setI", "SR-PS-SKEW-123:setI", "SR-PS-SKEW-124:setI", "SR-PS-SKEW-125:setI", "SR-PS-SKEW-126:setI", "SR-PS-SKEW-127:setI", "SR-PS-SKEW-131:setI", "SR-PS-SKEW-132:setI", "SR-PS-SKEW-133:setI", "SR-PS-SKEW-134:setI", "SR-PS-SKEW-135:setI", "SR-PS-SKEW-136:setI", "SR-PS-SKEW-137:setI", "SR-PS-SKEW-141:setI", "SR-PS-SKEW-142:setI", "SR-PS-SKEW-143:setI", "SR-PS-SKEW-144:setI", "SR-PS-SKEW-145:setI", "SR-PS-SKEW-146:setI", "SR-PS-SKEW-147:setI", "SR-PS-SKEW-151:setI", "SR-PS-SKEW-152:setI", "SR-PS-SKEW-153:setI", "SR-PS-SKEW-154:setI", "SR-PS-SKEW-155:setI", "SR-PS-SKEW-156:setI", "SR-PS-SKEW-157:setI", "SR-PS-SKEW-161:setI", "SR-PS-SKEW-162:setI", "SR-PS-SKEW-163:setI", "SR-PS-SKEW-164:setI", "SR-PS-SKEW-165:setI", "SR-PS-SKEW-166:setI", "SR-PS-SKEW-167:setI", "SR-PS-SKEW-171:setI", "SR-PS-SKEW-172:setI", "SR-PS-SKEW-173:setI", "SR-PS-SKEW-174:setI", "SR-PS-SKEW-175:setI", "SR-PS-SKEW-176:setI", "SR-PS-SKEW-177:setI", "SR-PS-SKEW-181:setI", "SR-PS-SKEW-182:setI", "SR-PS-SKEW-183:setI", "SR-PS-SKEW-184:setI", "SR-PS-SKEW-185:setI", "SR-PS-SKEW-186:setI", "SR-PS-SKEW-187:setI", "SR-PS-SKEW-191:setI", "SR-PS-SKEW-192:setI", "SR-PS-SKEW-193:setI", "SR-PS-SKEW-194:setI", "SR-PS-SKEW-195:setI", "SR-PS-SKEW-196:setI", "SR-PS-SKEW-197:setI", "SR-PS-SKEW-201:setI", "SR-PS-SKEW-202:setI", "SR-PS-SKEW-203:setI", "SR-PS-SKEW-204:setI", "SR-PS-SKEW-205:setI", "SR-PS-SKEW-206:setI", "SR-PS-SKEW-207:setI", "SR-PS-SKEW-211:setI", "SR-PS-SKEW-212:setI", "SR-PS-SKEW-213:setI", "SR-PS-SKEW-214:setI", "SR-PS-SKEW-215:setI", "SR-PS-SKEW-216:setI", "SR-PS-SKEW-217:setI", "SR-PS-SKEW-221:setI", "SR-PS-SKEW-222:setI", "SR-PS-SKEW-223:setI", "SR-PS-SKEW-224:setI", "SR-PS-SKEW-225:setI", "SR-PS-SKEW-226:setI", "SR-PS-SKEW-227:setI", "SR-PS-SKEW-231:setI", "SR-PS-SKEW-232:setI", "SR-PS-SKEW-233:setI", "SR-PS-SKEW-234:setI", "SR-PS-SKEW-235:setI", "SR-PS-SKEW-236:setI", "SR-PS-SKEW-237:setI", "SR-PS-SKEW-241:setI", "SR-PS-SKEW-242:setI", "SR-PS-SKEW-243:setI", "SR-PS-SKEW-244:setI", "SR-PS-SKEW-245:setI", "SR-PS-SKEW-246:setI", "SR-PS-SKEW-247:setI", "SR-RF2-LLRF:setGapVoltage", "SR-RF2-LLRF:setStationPhase", "SR-RF3-LLRF:setGapVoltage", "SR-RF3-LLRF:setStationPhase", "SR-PS-DMB09-Q1:setI", "SR-PS-DMB09-Q2:setI", "SR-PS-DMB09-Q3:setI", "SR-PS-DMB25-Q1:setI", "SR-PS-DMB25-Q2:setI", "SR-PS-DMB25-Q3:setI", "SR-PS-DMB41-Q1:setI", "SR-PS-DMB41-Q2:setI", "SR-PS-DMB41-Q3:setI", "SR-PS-DMB09-HC1:setI", "SR-PS-DMB09-HC2:setI", "SR-PS-DMB09-VC1:setI", "SR-PS-DMB09-VC2:setI", "SR-PS-DMB25-HC1:setI", "SR-PS-DMB25-HC2:setI", "SR-PS-DMB25-VC1:setI", "SR-PS-DMB25-VC2:setI", "SR-PS-DMB41-HC1:setI", "SR-PS-DMB41-HC2:setI", "SR-PS-DMB41-VC1:setI", "SR-PS-DMB41-VC2:setI", "SR-ID-IU22-05:setGap", "SR-ID-IU22A-09:setGap", "SR-ID-IU22B-09:setGap", "SR-ID-IUT22-21:setGap", "SR-ID-IU22-23:setGap", "SR-ID-IU22A-25:setGap", "SR-ID-IU22B-25:setGap", "SR-ID-EPU48A-41:setGap", "SR-ID-EPU48A-41:setPhase", "SR-ID-EPU48B-41:setGap", "SR-ID-EPU48B-41:setPhase", "SR-ID-EPU46-45:setGap", "SR-ID-EPU46-45:setPhase", "SR-ID-IUT22-21:getGapTaper", "SR-ID-EPU48PS-41:setGap", "SR-ID-IUT22-21:setGapMode", "SR-ID-IU22-05:gapMotorOff", "SR-ID-IU22A-09:gapMotorOff", "SR-ID-IU22B-09:gapMotorOff", "SR-ID-IUT22-21:gapMotorOff", "SR-ID-IU22-23:gapMotorOff", "SR-ID-IU22A-25:gapMotorOff", "SR-ID-IU22B-25:gapMotorOff", "SR-ID-EPU48A-41:gapMotorOff", "SR-ID-EPU48B-41:gapMotorOff", "SR-ID-EPU46-45:gapMotorOff", "SR-ID-EPU48A-41:phaseMotorOff", "SR-ID-EPU48B-41:phaseMotorOff", "SR-ID-EPU46-45:phaseMotorOff", "SR-ID-IU22-05:setECMode", "SR-ID-IU22A-09:setECMode", "SR-ID-IU22B-09:setECMode", "SR-ID-IUT22-21:setECMode", "SR-ID-IU22-23:setECMode", "SR-ID-IU22A-25:setECMode", "SR-ID-IU22B-25:setECMode", "SR-ID-EPU48A-41:setECMode", "SR-ID-EPU48B-41:setECMode", "SR-ID-EPU46-45:setECMode", "SR-DI-FOFB-H:setStatus", "SR-DI-FOFB-V:setStatus", "IGPF:TPSX:FBCTRL", "IGPF:TPSY:FBCTRL", "TPS-SR-022:bpm3:ilk:enabled", "SR-DI-ANGLE-ILK:StatusX", "SR-DI-ANGLE-ILK:StatusY", "SR-DI-RF-FB:setStatus", "SR-ID-EPU48-TFF:status", "SR-ID-EPU48-CFF:status", "SR-ID-EPU46-TFF:status", "SR-ID-EPU46-CFF:status", "TI-INJ-PROC:TopupHiLowStart", "TI-INJ-PROC:setBucketAddressStart", "TI-INJ-PROC:setBucketAddressLast", "TI-INJ-PROC:setBucketAddressStep", "TI-INJ-PROC:setPreCycle", "TI-INJ-PROC:setPostCycle", "TI-INJ-PROC:setBeamCurrentTopupHi", "TI-INJ-PROC:setBeamCurrentTopupLo", "TI-INJ-PROC:setSingleBunchAddr", "TI-INJ-PROC:setSingleInjCycle", "TI-INJ-PROC:setSingleBeamCurrent", "LI:controlState0", "TI-INJ-PROC:trig-BRAC-ONOFF", "SR:controlState0", "SR-DI-XPC-40:cam:AcquireTime", "SR-DI-XPC-40:cam:Gain"] ("PV list")
  n1 = Array Size(array=w1) -> (size(s)=→"size(s)":i32)
  n2 = call-poly <userlib>:"CaLabGet.vi"("PV Names"=w1, "NoMDEL(F)"=FALSE) -> ("1rst Value (string)"=w8:string[], "Status"=→"Status":bool, "Error out"=→"Error out":errorcluster)  [unwired: 7 in, 4 out]
  "1rst Value (string)" <- w8
  n3 = Array Size(array=w8) -> (size(s)=→"size(s) 2":i32)
  n4 = for {
    tunnel: w8 -> [w15] mode=indexing
    tunnel: [w14] -> w7 mode=indexing
    tunnel: [w13] -> w5 mode=indexing if=w12
    i -> [w13]
    n5 = Empty String/Path?(string/path=w15) -> (empty?=w12:bool)
    n6 = Boolean To (0,1)(Boolean=w12) -> (0, 1=w14:i16)
    "Numeric Control" <- w13
  }
  "Array" <- w5
  n7 = Empty Array?(array=w5) -> (empty?=w4:bool)
  "empty?" <- w4
  n8 = Add Array Elements(numeric array=w7) -> (sum=→"sum":i16)
  n9 = case shown="False" w4 {
    tunnel: w1 -> [w17 _]
    tunnel: w5 -> [w16 _]
    frame False {
      n10 = for {
        tunnel: w17 -> [w23]
        tunnel: w16 -> [w22] mode=indexing
        tunnel: [w21] -> w19 mode=indexing
        i -> [w20]
        n11 = Index Array(array=w23, index=w22) -> (element=w21:string)
        "Numeric Control 2" <- w20
      }
      "Array 2" <- w19
      n12 = call-poly <userlib>:"CaLabGet.vi"("PV Names"=w19) -> ("1rst Value (string)"=→"1rst Value (string) 2":string[])  [unwired: 8 in, 6 out]
    }
    frame True {
      n13 = One Button Dialog(message="All PVs OK", button name ("OK")="YES!!") -> ()  [unwired: 1 out]
    }
  }
